vi "Dead_Zone.vi"(1 "Range":dbl=1.0 min=0.0 step=0.25, 2 "Slope of 1":bool, 3 "Dead Zone and Limits":cluster{dbl, dbl}(slide)={0.05, 1.0} scale=0.0..1.0, 4 "Input":dbl step=0.01) -> (0 "Output":dbl)   [LabVIEW 2014]
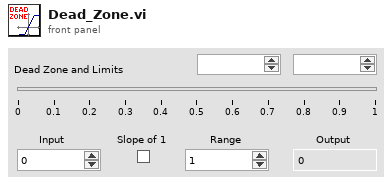
[diagram p1: front panel]
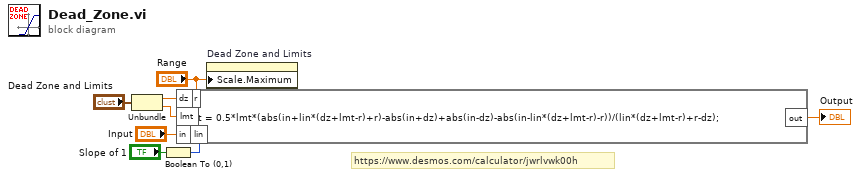
[diagram p0: block diagram]
diagram:
  # "https://www.desmos.com/calculator/jwrlvwk00h"
  n1 = Unbundle("Dead Zone and Limits") -> (w5:dbl, w4:dbl)
  n2 = Boolean To (0,1)(Boolean="Slope of 1") -> (0, 1=w2:i16)
  n3 = formula code="out = 0.5*lmt*(abs(in+lin*(dz+lmt-r)+r)-abs(in+dz)+abs(in-dz)-abs(in-lin*(dz+lmt-r)-r))/(lin*(dz+lmt-r)+r-dz);"("dz"=w5, "lmt"=w4, "in"="Input", "lin"=w2, "r"="Range") -> ("out"=→"Output":dbl)
  n4 = property on="Dead Zone and Limits" class="Slide (strict)"("Scale.Maximum"="Range") -> ()  [unwired: 2 in, 2 out]
